vi "RPC Server (test).vi"() -> ()   [LabVIEW 2020]
uses:
  External/JSON-RPC/Classes/Server/Add Response (Result from Request).vi
  External/JSON-RPC/Classes/Server/Add Response (Server Error from Request).vi
  External/JSON-RPC/Classes/Server/Add Response (Internal Error from Request).vi
  External/JSON-RPC/Classes/Server/Send Request (Sync).vi
  Realization/RPC.lvlib
  External/JSON-RPC/Classes/Server/JSONRPC Server.lvclass
panel:
  out "header":string
  out "request":string
  out "response":string
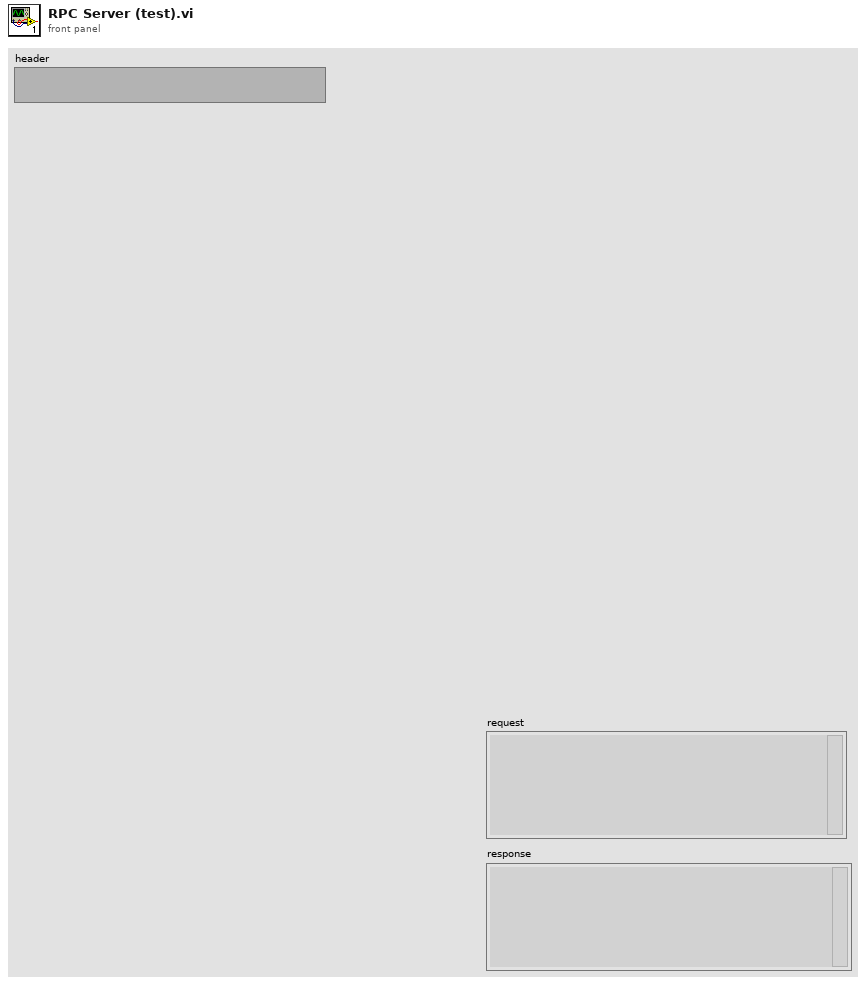
[diagram p1: front panel]
types:
  T1 = enum16{"Standard", "Buffered", "CRLF", "Immediate"}
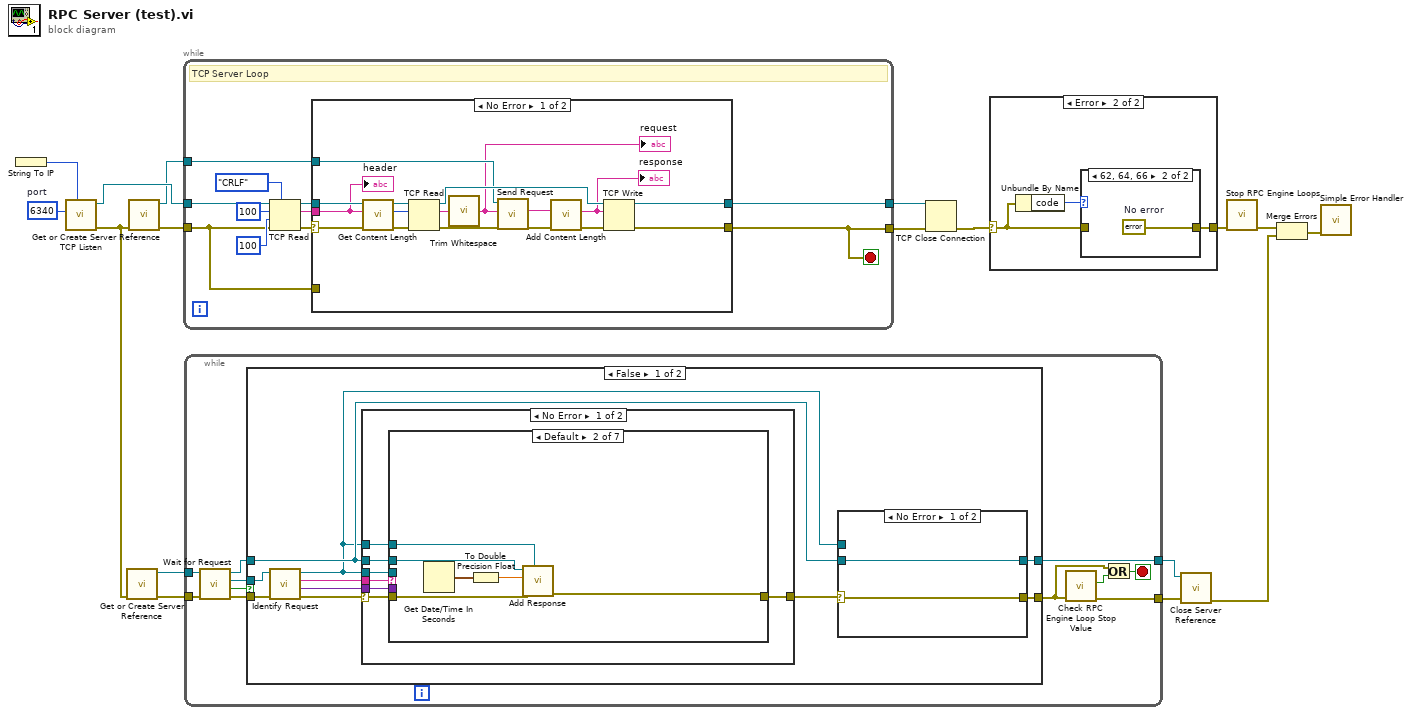
[diagram p0: block diagram]
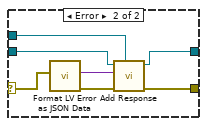
[diagram p2: hidden frame]
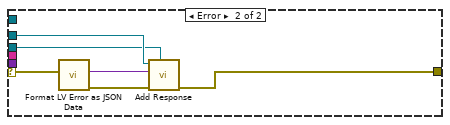
[diagram p9: hidden frame]
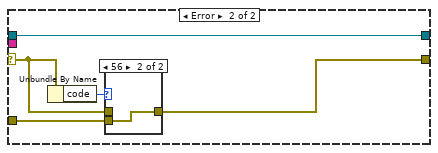
[diagram p13: hidden frame]
diagram:
  w15 = u16 6340  # port
  n1 = String To IP() -> (0:w14:u32)  [unwired: 1 in]
  n2 = call <vilib>:"TCP Listen.vi"("net address"=w14, "port"=w15) -> ("error out"=w3:errorcluster, "connection ID"=w12:refnum<k5>)  [unwired: 5 in, 3 out]
  n3 = call "Get or Create Server Reference.vi"("error in (no error)"=w3) -> ("error out"=w8:errorcluster, "Server Out"=w1:refnum<class "JSONRPC Server.lvclass">)  [unwired: 9 in]
  n4 = call "Get or Create Server Reference.vi"("error in (no error)"=w3) -> ("error out"=w11:errorcluster, "Server Out"=w10:refnum<class "JSONRPC Server.lvclass">)  [unwired: 9 in]
  n5 = while {
    tunnel: [w18] -> w16
    tunnel: [w25] -> w17
    tunnel: w12 -> [w21]
    tunnel: w11 -> [w22]
    tunnel: w10 -> [w19]
    stop <- w18 stop-if-true
    # "TCP Server Loop"
    n6 = TCP Read(connection ID=w21, bytes to read=100, error in (no error)=w22, 7:T1."CRLF" ("mode (standard)"), 9:100 ("timeout ms (25000)")) -> (connection ID out=w26:refnum<k5>, data out=w20:string, error out=w24:errorcluster)
    n7 = case shown="No Error" w24 {
      selector: w24 -> [w44 w48]
      tunnel: [w38 w46] -> w18
      tunnel: w22 -> [_ w47]
      tunnel: [w39 w45] -> w25
      tunnel: w26 -> [w42 w45]
      tunnel: w20 -> [w41 _]
      tunnel: w19 -> [w35 _]
      frame No Error {
        n8 = call "Get Content Length.vi"("error in (no error)"=w44, "header"=w41) -> ("error out"=w43:errorcluster, "content length"=w40:i32)  [unwired: 8 in]
        n9 = TCP Read(connection ID=w42, bytes to read=w40, error in (no error)=w43) -> (connection ID out=w37:refnum<k5>, data out=w30:string, error out=w36:errorcluster)  [unwired: 2 out]
        n10 = call <vilib>:"Trim Whitespace.vi"("string"=w30) -> ("trimmed string"=w29:string)  [unwired: 1 in]
        "request" <- w29
        n11 = call-poly "Send Request.vi"("error in (no error)"=w36, "JSON Request String"=w29, "JSONRPC Server in"=w35) -> ("error out"=w34:errorcluster, "JSON Response String"=w31:string)  [unwired: 6 in, 1 out]
        n12 = call "Add Content Length.vi"("error in (no error)"=w34, "JSON Response String in"=w31) -> ("error out"=w33:errorcluster, "JSON Response String out"=w32:string)  [unwired: 8 in]
        "response" <- w32
        n13 = TCP Write(connection ID=w37, data in=w32, error in (no error)=w33) -> (connection ID out=w39:refnum<k5>, error out=w38:errorcluster)  [unwired: 1 in, 1 out]
        "header" <- w41
      }
      frame Error {
        n14 = Unbundle By Name(w48) -> ("code"=w49:i32)
        n15 = case shown="56" w49 {
          tunnel: w48 -> [w50 _]
          tunnel: w47 -> [_ w51]
          tunnel: [w50 w51] -> w46
          frame Default {
          }
          frame 56 {
          }
        }
      }
    }
  }
  n16 = while {
    tunnel: w8 -> [w62]
    tunnel: w1 -> [w61]
    tunnel: [w56] -> w7
    tunnel: [w55] -> w6
    stop <- w52 stop-if-true
    n17 = call "Wait for Request.vi"("error in (no error)"=w62, "Server in"=w61) -> ("error out"=w60:errorcluster, "timed out?"=w57:bool, "Request"=w59:refnum<class "Request.lvclass">, "Server out"=w58:refnum<class "JSONRPC Server.lvclass">)  [unwired: 6 in]
    n18 = case shown="False" w57 {
      tunnel: w60 -> [w66 w108]
      tunnel: w59 -> [w72 _]
      tunnel: w58 -> [w64 w107]
      tunnel: [w69 w108] -> w53
      tunnel: [w68 w107] -> w55
      frame False {
        n19 = call "Identify Request.vi"("error in (no error)"=w66, "Request in"=w72) -> ("error out"=w67:errorcluster, "params"=w71:variant, "method"=w65:string, "Request out"=w63:refnum<class "Request.lvclass">)  [unwired: 5 in, 1 out]
        n20 = case shown="No Error" w67 {
          selector: w67 -> [w86 w106]
          tunnel: w71 -> [w83 _]
          tunnel: w64 -> [w88 w104]
          tunnel: w63 -> [w87 w103]
          tunnel: [w85 w101] -> w70
          tunnel: w65 -> [w84 _]
          tunnel: w63 -> [w82 _]
          frame No Error {
            n21 = case shown="Default" w84 {
              tunnel: w88 -> [_ w94 _ _ _ _ _]
              tunnel: w87 -> [_ _ _ _ _ _ _]
              tunnel: w86 -> [w89 w95 w96 w97 w98 w99 w100]
              tunnel: [w89 w92 w96 w97 w98 w99 w100] -> w85
              tunnel: w83 -> [_ _ _ _ _ _ _]
              tunnel: w82 -> [_ w93 _ _ _ _ _]
              frame "rpc_server_init" {
              }
              frame Default {
                n22 = Get Date/Time In Seconds() -> (seconds since 1Jan1904=w90:timestamp)
                n23 = To Double Precision Float(number=w90) -> (double precision float=w91:dbl)
                n24 = call-poly "Add Response.vi"("Request"=w93, "error in (no error)"=w95, "JSON Value in"=w91, "Server in"=w94) -> ("error out"=w92:errorcluster)  [unwired: 5 in, 2 out]
              }
              frame "rpc_server_dispatch" {
              }
              frame "rpc_server_launch_module" {
              }
              frame "rpc_server_shutdown_module" {
              }
              frame "rpc_server_broadcast" {
              }
              frame "rpc_server_shutdown" {
              }
            }
          }
          frame Error {
            n25 = call "Format LV Error as JSON Data.vi"("error in"=w106) -> ("error out"=w105:errorcluster, "Error Value out"=w102:variant)  [unwired: 9 in]
            n26 = call-poly "Add Response.vi"("Request"=w103, "error in (no error)"=w105, "data"=w102, "Server in"=w104) -> ("error out"=w101:errorcluster)  [unwired: 5 in, 2 out]
          }
        }
        n27 = case shown="No Error" w70 {
          selector: w70 -> [w74 w79]
          tunnel: [w74 w78] -> w69
          tunnel: w64 -> [w73 w76]
          tunnel: [w73 w77] -> w68
          tunnel: w63 -> [_ w75]
          frame No Error {
          }
          frame Error {
            n28 = call "Format LV Error as JSON Data.vi"("error in"=w79) -> ("error out"=w81:errorcluster, "Error Value out"=w80:variant)  [unwired: 9 in]
            n29 = call-poly "Add Response.vi"("Request"=w75, "error in (no error)"=w81, "data"=w80, "Server in"=w76) -> ("error out"=w78:errorcluster, "Server out"=w77:refnum<class "JSONRPC Server.lvclass">)  [unwired: 5 in, 1 out]
          }
        }
      }
      frame True {
      }
    }
    n30 = call "Check RPC Engine Loop Stop Value.vi"("error in (no error)"=w53) -> ("error out"=w56:errorcluster, "stopped?"=w54:bool)  [unwired: 9 in]
    n31 = Or(x=w53, y=w54) -> (x .or. y?=w52:bool)
  }
  n32 = TCP Close Connection(connection ID=w17, error in (no error)=w16) -> (error out=w13:errorcluster)  [unwired: 2 out]
  n33 = case shown="Error" w13 {
    selector: w13 -> [w109 w111]
    tunnel: [w109 w110] -> w9
    frame No Error {
    }
    frame Error {
      n34 = Unbundle By Name(w111) -> ("code"=w112:i32)
      n35 = case shown="62, 64, 66" w112 {
        tunnel: w111 -> [w113 _]
        tunnel: [w113 w114] -> w110
        frame Default {
        }
        frame 62, 64, 66 {
          w114 = errorcluster {"status"=FALSE, "code"=0, "source"=""}  # No error
        }
      }
    }
  }
  n36 = call "Close Server Reference.vi"("error in (no error)"=w7, "Server in"=w6) -> ("error out"=w2:errorcluster)  [unwired: 9 in]
  n37 = call "Stop RPC Engine Loops.vi"("error in (no error)"=w9) -> ("error out"=w5:errorcluster)  [unwired: 10 in]
  n38 = Merge Errors(w5, w2) -> (w4:errorcluster)
  n39 = call <vilib>:"Simple Error Handler.vi"("error in (no error)"=w4) -> ()  [unwired: 1 in, 8 out]
